vi "MAT_Body.vi"(6 "byte order":T1(ring), 8 "Dimensions":i32[](array[numeric]), 10 "Imag":dbl[](array[numeric]), 11 "Real":dbl[](array[numeric])) -> (2 "String Out":string, 3 "length":i32)   [LabVIEW 2022 SP3]
uses:
  Subs/miDataType.ctl
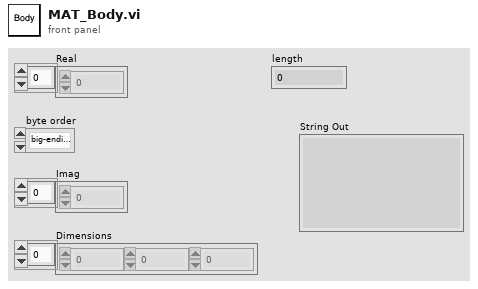
[diagram p1: front panel]
types:
  T1 = enum16{"big-endian, network order", "native, host order", "little-endian"}
  T2 = cluster{"data":string, "Dimensions":i32[], "payload":string, "btns":cluster{"complex":bool, "global":bool, "logical":bool}}
  T3 = typedef "miDataType.ctl" = enum16{"illegal", "miINT8", "miUINT8", "miINT16", "miUINT16", "miINT32", "miUINT32", "miSINGLE", "--", "miDOUBLE", "---", "----", "miINT64", "miUINT64", "miMATRIX", "miCOMPRESSED", "miUTF8", "miUTF16", "miUTF32", "udefined"}
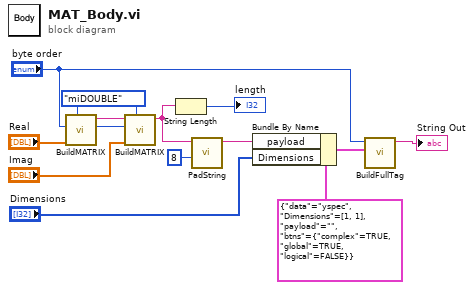
[diagram p0: block diagram]
diagram:
  w2 = miDataType."miDOUBLE" ("Data Type")
  n1 = call "BuildMATRIX.vi"("Data Type"=w2, "data"="Real", "byte order"="byte order") -> ("String out"=w1:string)  [unwired: 8 in]
  n2 = call "BuildMATRIX.vi"("Data Type"=w2, "data"="Imag", "byte order"="byte order", "String in"=w1) -> ("String out"=w12:string)  [unwired: 7 in]
  n3 = String Length(string=w12) -> (length=→"length":i32)
  n4 = call "PadString.vi"("size"=8, "data"=w12) -> ("String"=w13:string)  [unwired: 9 in]
  n5 = Bundle By Name(cluster=T2 {"data"="yspec", "Dimensions"=[1, 1], "payload"="", "btns"={"complex"=TRUE, "global"=TRUE, "logical"=FALSE}}, "payload"=w13, "Dimensions"="Dimensions") -> (w8:T2)
  n6 = call "BuildFullTag.vi"("Cluster"=w8, "byte order"="byte order") -> ("String Out"=→"String Out":string)  [unwired: 9 in]
